vi "Logger Ready.vi"(8 "error in (no error)":errorcluster, 10 "Logger Ready":T1, 11 "Historian Logger in":refnum<class "Historian Logger.lvclass">) -> (0 "error out":errorcluster, 3 "Historian Logger out":refnum<class "Historian Logger.lvclass">)   [LabVIEW 2020, in "VolatusHistorian.lvlib" / "Historian Logger.lvclass"]
uses:
  Historian Logger.lvclass
  Historian Logger.lvclass/Historian Logger.ctl
  VolatusData/Logger State.ctl
  VolatusData/VolatusData.lvlib
  VolatusData/Logger Ready.ctl
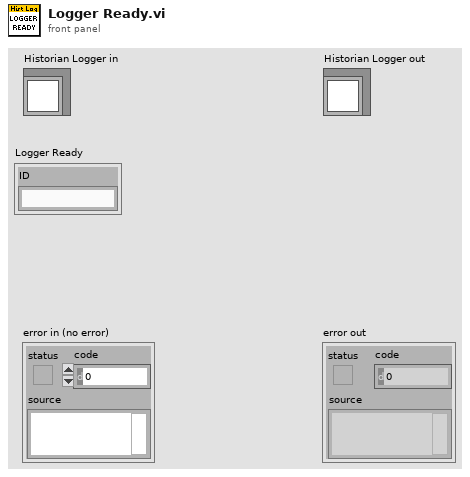
[diagram p1: front panel]
types:
  T1 = typedef "VolatusData.lvlib/Logger Ready.ctl" = cluster{"ID":string}
  T2 = typedef "VolatusData.lvlib/Logger State.ctl" = enum16{"Unknown", "Idle", "Preparing", "Ready", "Logging", "Stopping"}
  T3 = typedef "VolatusHistorian.lvlib/Historian Logger.lvclass/Group Info.ctl" = cluster{"Buffer":refnum<class "Group Buffer DBL.lvclass">, "Logger":refnum<class "MessageQ.lvclass">, "Group":refnum<class "Group DBL.lvclass">, "Last Timestamp":dbl, "State":T2}
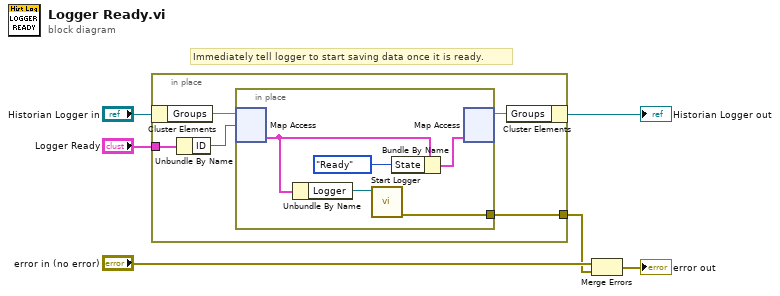
[diagram p0: block diagram]
diagram:
  # "Immediately tell logger to start saving data once it is ready."
  n1 = in-place {
    in-place-border: "Logger Ready" -> [w11]
    in-place-border: [w7] -> w1
    n2 = in-place-cluster #1("Historian Logger in") -> ("Groups"=w10:map{string, T3})
    n3 = Unbundle By Name(w11) -> ("ID"=w9:string)
    n4 = in-place {
      in-place-border: [w12] -> w7
      n5 = in-place-map #2(w10, w9) -> (w14:T3)  [unwired: 1 in, 1 out]
      n6 = Unbundle By Name(w14) -> ("Logger"=w13:refnum<class "MessageQ.lvclass">)
      n7 = call "Start Logger.vi"("MsgQ in"=w13) -> ("error out"=w12:errorcluster)  [unwired: 9 in, 1 out]
      n8 = Bundle By Name(cluster=w14, "State"=Logger_State."Ready") -> (w15:T3)
      n9 = in-place-map #2(w15) -> (w8:map{string, T3})  [unwired: 1 in, 2 out]
    }
    n10 = in-place-cluster #1("Groups"=w8) -> (→"Historian Logger out":refnum<class "Historian Logger.lvclass">)
  }
  n11 = Merge Errors("error in (no error)", w1) -> (→"error out":errorcluster)
